vi "SimpleExampleOOP(MM).vi"() -> ()   [LabVIEW 2013]
uses:
  StellarNetSpecAcquisitionClass/StellarNetSpecAcquisition.lvclass
  StellarNetSpectrometerClass/StellarNetSpectrometer.lvclass
panel:
  in  "Boolean":bool
  in  "Settings":T1={"Integration Time (ms)"=80, "Temp  Compensation "=FALSE, "Optical Smoothing Level"=0, "Number of Scans to Average"=1, "Digitizer Clock Rate Setting"=3}
  out "Spectrum":sgl[](graph)
  out "OK":bool
  in  "stop":bool
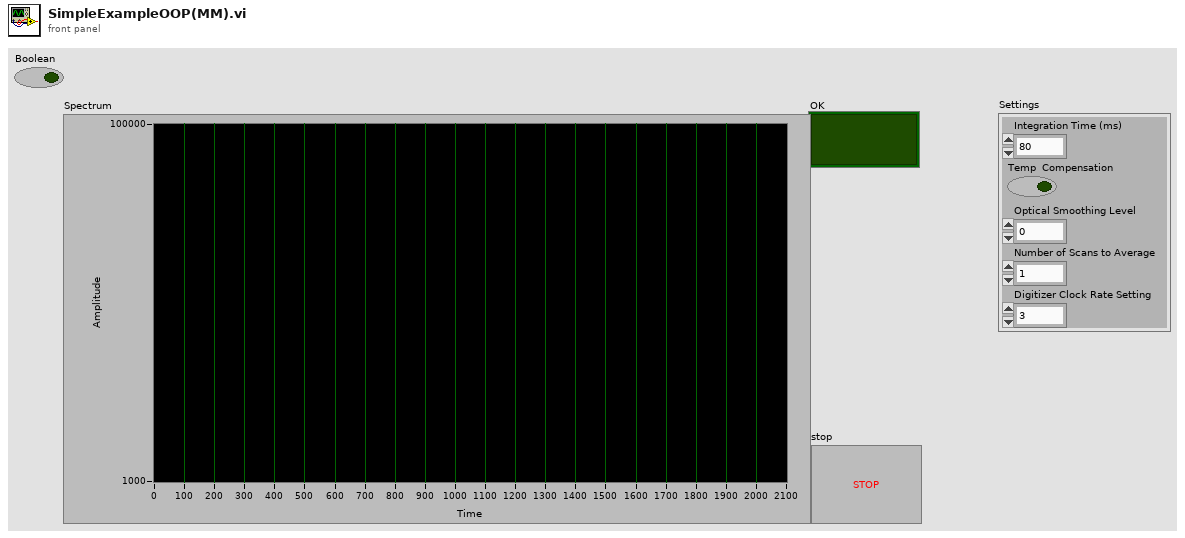
[diagram p1: front panel]
types:
  T1 = cluster{"Integration Time (ms)":i32, "Temp  Compensation ":bool, "Optical Smoothing Level":i32, "Number of Scans to Average":i32, "Digitizer Clock Rate Setting":i32}
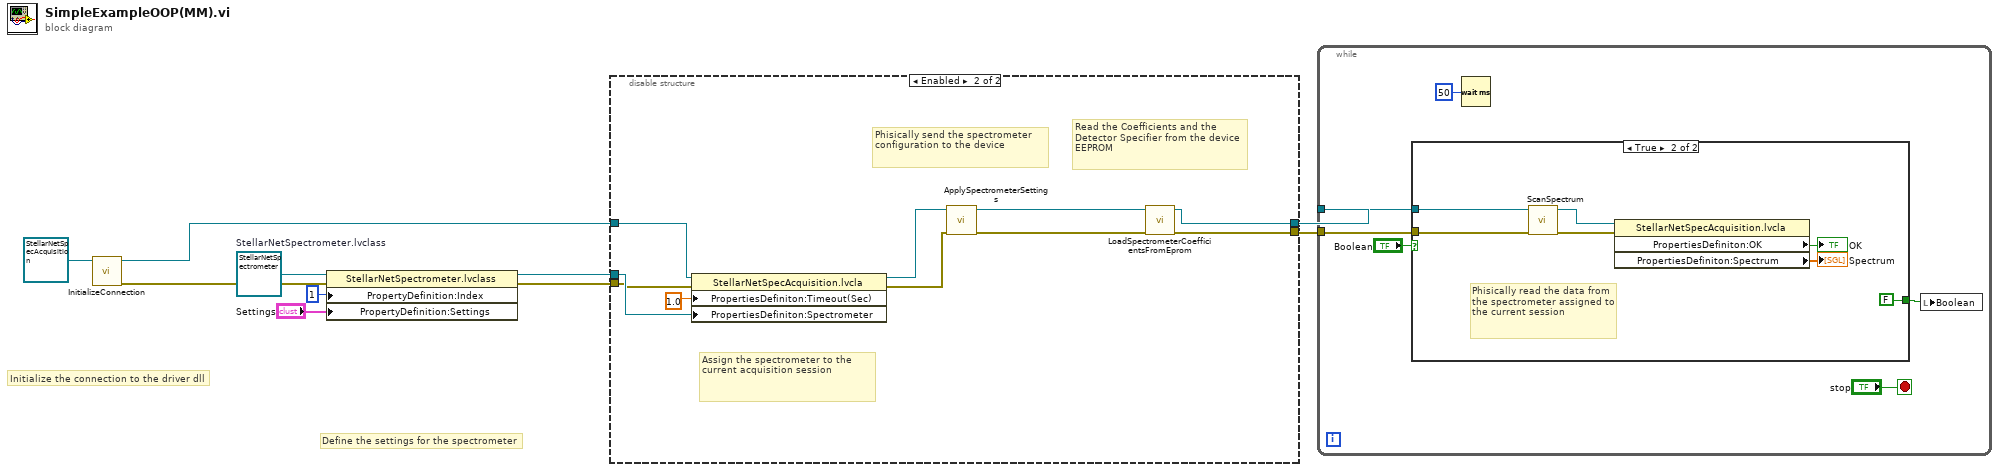
[diagram p0: block diagram]
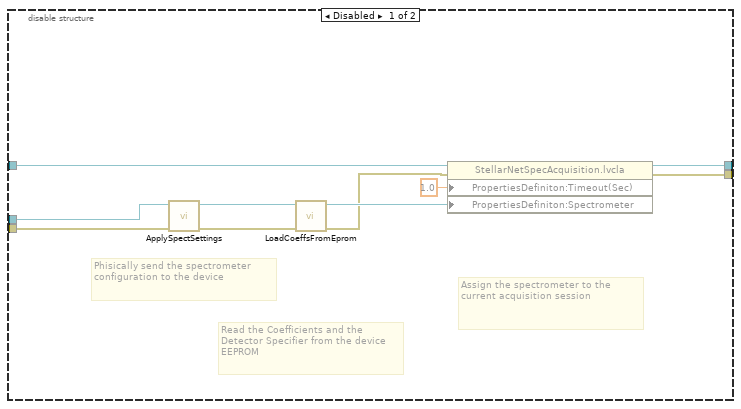
[diagram p2: hidden frame]
diagram:
  w10 = refnum<class "StellarNetSpectrometer.lvclass"> refnum  # StellarNetSpectrometer.lvclass
  # "Initialize the connection to the driver dll"
  # "Define the settings for the spectrometer"
  n1 = call-dynamic "InitializeConnection.vi"("StellarNetSpecAcquisition in"=refnum<class "StellarNetSpecAcquisition.lvclass"> refnum ("StellarNetSpecAcquisition.lvclass")) -> ("error out"=w2:errorcluster, "StellarNetSpecAcquisition out"=w3:refnum<class "StellarNetSpecAcquisition.lvclass">)  [unwired: 9 in]
  n2 = property class="StellarNetSpectrometer.lvclass"(reference=w10, error in=w2, "PropertyDefinition:Index"=u32 1 ("Index"), "PropertyDefinition:Settings"="Settings") -> (reference out=w6:refnum<class "StellarNetSpectrometer.lvclass">, error out=w5:errorcluster)
  n3 = disable-structure shown="Enabled" {
    disable-tunnel: [w20 w22] -> w8
    disable-tunnel: [w19 w21] -> w7
    disable-tunnel: w6 -> [w18 w24]
    disable-tunnel: w5 -> [w17 w23]
    disable-tunnel: w3 -> [w16 w25]
    frame Disabled {
      # "Assign the spectrometer to the current acquisition session"
      # "Read the Coefficients and the Detector Specifier from the device EEPROM"
      # "Phisically send the spectrometer configuration to the device"
      n4 = call-dynamic "ApplySpectSettings.vi"("error in"=w17, "StellarNetSpectrometer in"=w18) -> ("error out"=w15:errorcluster, "StellarNetSpectrometer out"=w14:refnum<class "StellarNetSpectrometer.lvclass">)  [unwired: 8 in]
      n5 = call-dynamic "LoadCoeffsFromEprom.vi"("error in"=w15, "StellarNetSpectrometer in"=w14) -> ("error out"=w12:errorcluster, "StellarNetSpectrometer out"=w13:refnum<class "StellarNetSpectrometer.lvclass">)  [unwired: 8 in]
      n6 = property class="StellarNetSpecAcquisition.lvcla"(reference=w16, error in=w12, "PropertiesDefiniton:Timeout(Sec)"=1.0 ("Timeout(Sec)"), "PropertiesDefiniton:Spectrometer"=w13) -> (reference out=w19:refnum<class "StellarNetSpecAcquisition.lvclass">, error out=w20:errorcluster)
    }
    frame Enabled {
      # "Assign the spectrometer to the current acquisition session"
      # "Read the Coefficients and the Detector Specifier from the device EEPROM"
      # "Phisically send the spectrometer configuration to the device"
      n7 = property class="StellarNetSpecAcquisition.lvcla"(reference=w25, error in=w23, "PropertiesDefiniton:Timeout(Sec)"=1.0 ("Timeout(Sec)"), "PropertiesDefiniton:Spectrometer"=w24) -> (reference out=w27:refnum<class "StellarNetSpecAcquisition.lvclass">, error out=w28:errorcluster)
      n8 = call-dynamic "ApplySpectrometerSettings.vi"("error in (no error)"=w28, "StellarNetSpecAcquisition in"=w27) -> ("error out"=w30:errorcluster, "StellarNetSpecAcquisition out"=w29:refnum<class "StellarNetSpecAcquisition.lvclass">)  [unwired: 8 in]
      n9 = call-dynamic "LoadSpectrometerCoefficientsFromEprom.vi"("error in (no error)"=w30, "StellarNetSpecAcquisition in"=w29) -> ("error out"=w22:errorcluster, "StellarNetSpecAcquisition out"=w21:refnum<class "StellarNetSpecAcquisition.lvclass">)  [unwired: 8 in]
    }
  }
  n10 = while {
    tunnel: w8 -> [w36]
    tunnel: w7 -> [w35]
    stop <- "stop" stop-if-true
    n11 = case shown="True" "Boolean" {
      tunnel: w36 -> [_ w43]
      tunnel: w35 -> [_ w42]
      tunnel: [_ FALSE] -> w31
      frame False {
      }
      frame True {
        # "Phisically read the data from the spectrometer assigned to the current session"
        n12 = call-dynamic "ScanSpectrum.vi"("error in"=w43, "StellarNetSpecAcquisition in"=w42) -> ("error out"=w40:errorcluster, "StellarNetSpecAcquisition out"=w41:refnum<class "StellarNetSpecAcquisition.lvclass">)  [unwired: 8 in]
        n13 = property class="StellarNetSpecAcquisition.lvcla"(reference=w41, error in=w40) -> ("PropertiesDefiniton:OK"=→"OK":bool, "PropertiesDefiniton:Spectrum"=→"Spectrum":sgl[])  [unwired: 2 out]
      }
    }
    n14 = Wait (ms)(milliseconds to wait=u32 50) -> ()  [unwired: 1 out]
    n15 = local write "Boolean"(w31) -> ()
  }
